vi "IsEmpty.vi"(8 "error in":errorcluster, 10 "number":i32) -> (0 "error out":errorcluster)   [LabVIEW 2022 SP3, in "PCA9685.lvlib" / "PCA.lvclass"]
uses:
  PCA.lvclass
  PCA.lvclass/PCA.ctl
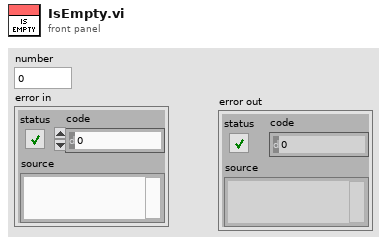
[diagram p1: front panel]
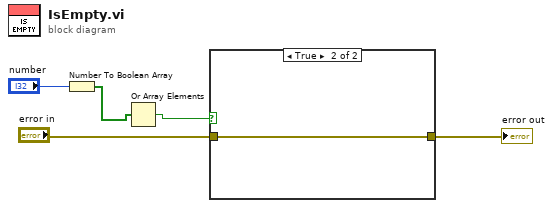
[diagram p0: block diagram]
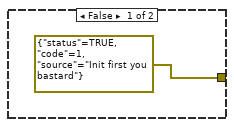
[diagram p2: hidden frame]
diagram:
  n1 = Number To Boolean Array(number="number") -> (Boolean array=w2:bool[])
  n2 = Or Array Elements(Boolean array=w2) -> (logical OR=w1:bool)
  n3 = case shown="True" w1 {
    tunnel: [errorcluster {"status"=TRUE, "code"=1, "source"="Init first you bastard"} ("error constant") w7] -> w5
    tunnel: "error in" -> [_ w7]
    frame False {
    }
    frame True {
    }
  }
  "error out" <- w5
